vi "CSMOMgr-Create CSMO.vi"(7 "Allowed Messages(Empty for all)":string[](array[string]), 8 "error in (no error)":errorcluster, 10 "Name(\"\" to use uuid) in":string, 11 "CSMOMgr":T1) -> (0 "error out":errorcluster, 2 "CSMO":T2, 3 "CSMOMgr out":T1)   [LabVIEW 2020, in "Communicable State Machine.lvlib"]
uses:
  Communicable State Machine.lvlib
  Def-CSMOMgr.ctl
  _CSMObj.ctl
  Priority Queue.lvclass
  _CSM_MODE.ctl
  _CSMObj-Data.ctl
  _CSM Status Change Event Data.ctl
  _CSMObj-ModeData.ctl
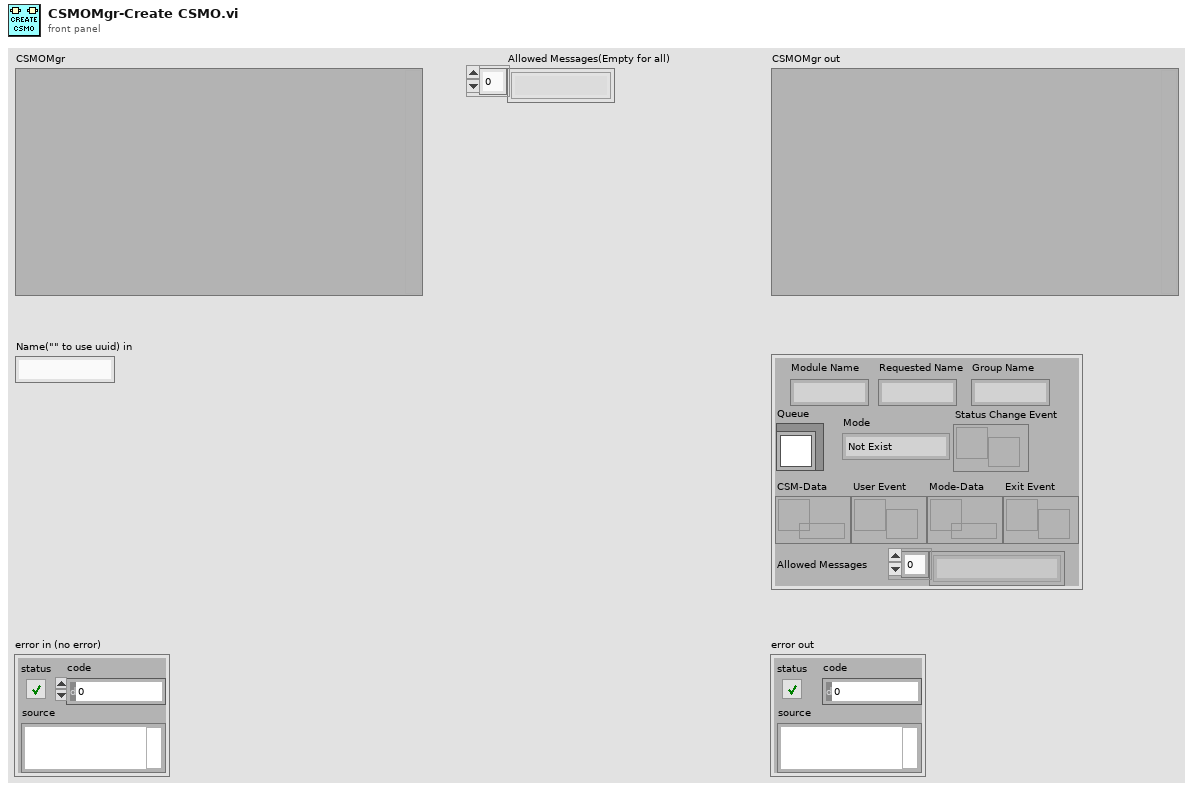
[diagram p1: front panel]
types:
  T1 = typedef "Communicable State Machine.lvlib/Def-CSMOMgr.ctl" = variant
  T2 = typedef "Communicable State Machine.lvlib/_CSMObj.ctl" = cluster{"Requested Name":string, "Module Name":string, "Mode":T3, "Queue":refnum<class "Priority Queue.lvclass">, "CSM-Data":refnum<data-value>, "User Event":refnum<user-event>, "Status Change Event":refnum<user-event>, "Allowed Messages":string[], "Mode-Data":refnum<data-value>, "Group Name":string, "Exit Event":refnum<user-event>}
  T3 = typedef "Communicable State Machine.lvlib/_CSM_MODE.ctl" = enum16{"Not Exist", "Stand Alone", "CSM", "Worker Agent", "Worker", "Chain", "Chain Node"}
  T4 = typedef "Communicable State Machine.lvlib/_CSM_NAME_REQUEST.ctl" = enum16{"Stand Alone CSM Request", "Normal CSM Request", "Agent Request", "Action Worker Request", "Chain Request", "Chain Node Request"}
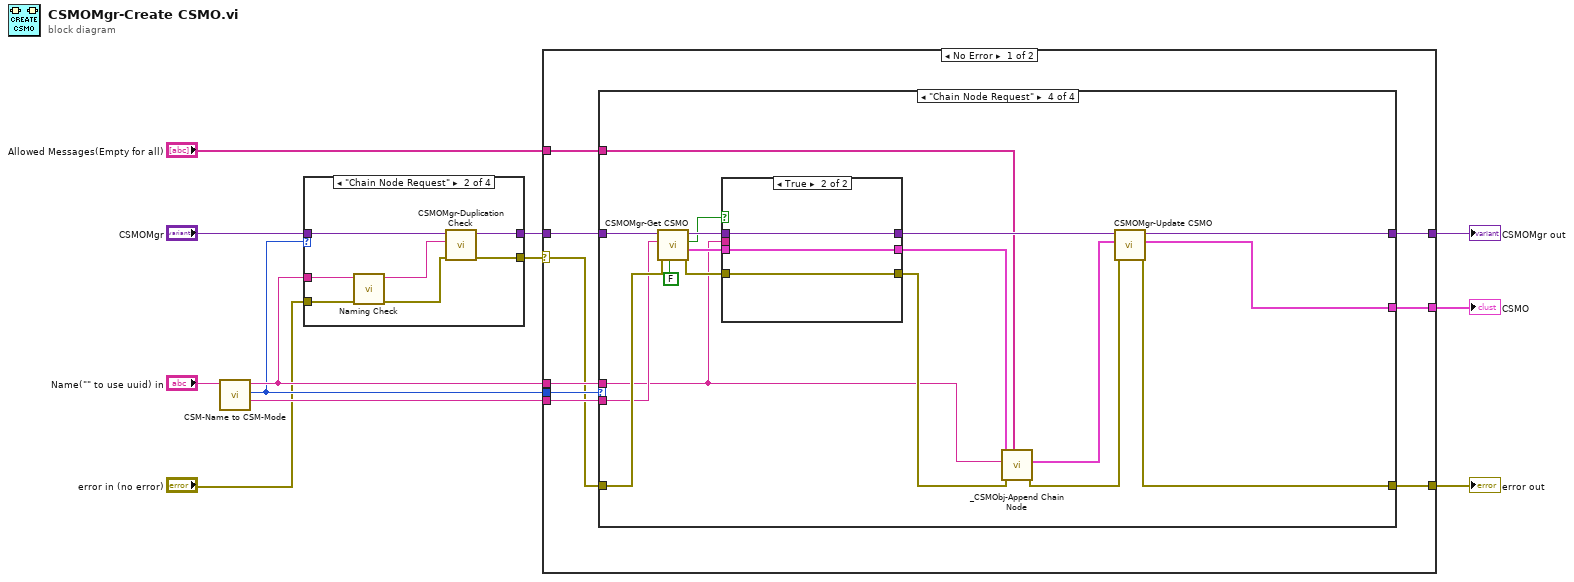
[diagram p0: block diagram]
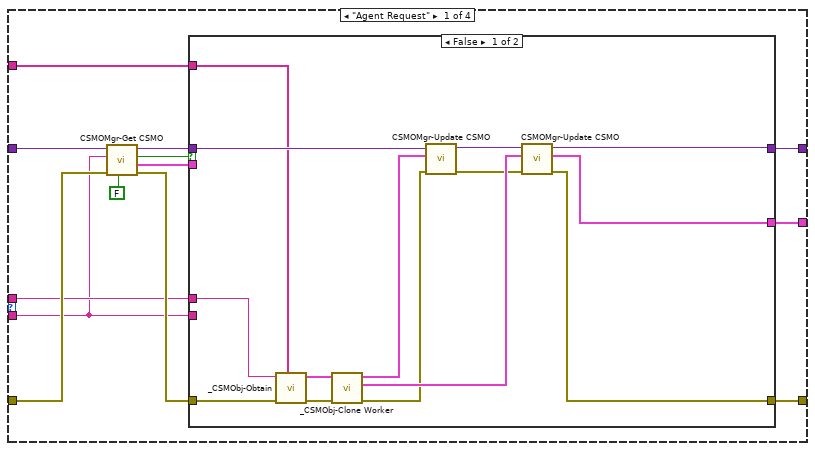
[diagram p2: hidden frame]
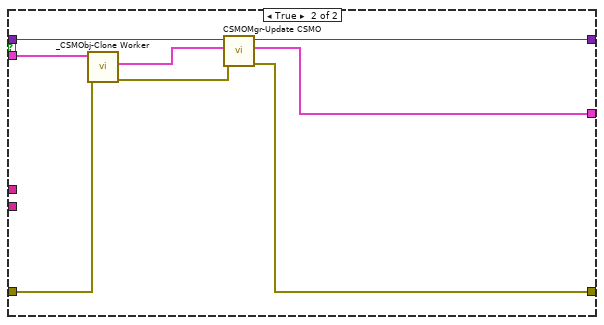
[diagram p3: hidden frame]
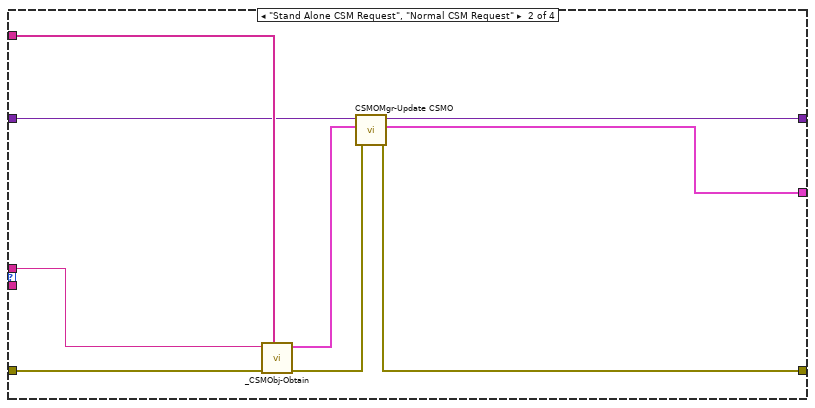
[diagram p4: hidden frame]
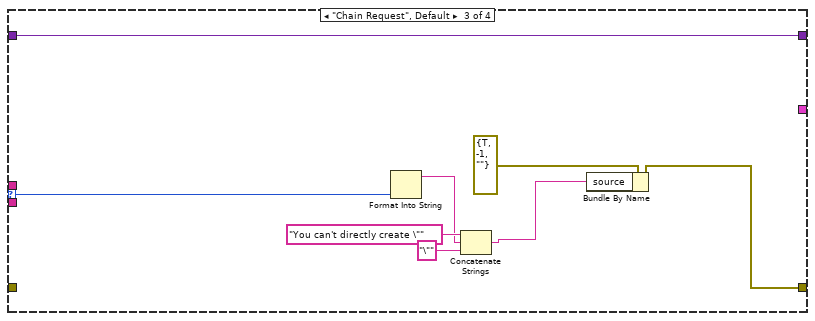
[diagram p5: hidden frame]
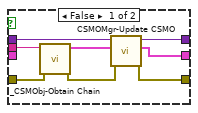
[diagram p6: hidden frame]
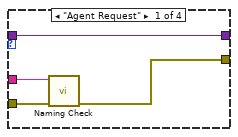
[diagram p8: hidden frame]
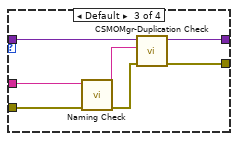
[diagram p9: hidden frame]
diagram:
  n1 = call "CSM-Name to CSM-Mode.vi"("String"="Name(\"\" to use uuid) in") -> ("ParentCSM Name"=w10:string, "CSM Mode"=w11:T4, "Requested Name"=w12:string)  [unwired: 8 in]
  n2 = case shown="\"Chain Node Request\"" w11 {
    tunnel: [w14 w20 w30 w32] -> w6
    tunnel: [w13 w18 w28 w31] -> w7
    tunnel: "CSMOMgr" -> [w14 w21 w26 w32]
    tunnel: "error in (no error)" -> [w15 w22 w25 w31]
    tunnel: w12 -> [w16 w23 w24 _]
    frame "Agent Request" {
      n3 = call "Naming Check.vi"("error in (no error)"=w15, "Name(\"\" to use uuid)"=w16) -> ("error out"=w13:errorcluster)  [unwired: 8 in, 1 out]
    }
    frame "Chain Node Request" {
      n4 = call "Naming Check.vi"("error in (no error)"=w22, "Name(\"\" to use uuid)"=w23) -> ("error out"=w17:errorcluster, "Name(dup)"=w19:string)  [unwired: 8 in]
      n5 = call "CSMOMgr-Duplication Check.vi"("Error in"=w17, "Queue Name"=w19, "CSMOMgr"=w21) -> ("Error out"=w18:errorcluster, "CSMOMgr out"=w20:T1)  [unwired: 7 in]
    }
    frame Default {
      n6 = call "Naming Check.vi"("error in (no error)"=w25, "Name(\"\" to use uuid)"=w24) -> ("error out"=w29:errorcluster, "Name(dup)"=w27:string)  [unwired: 8 in]
      n7 = call "CSMOMgr-Duplication Check.vi"("Error in"=w29, "Queue Name"=w27, "CSMOMgr"=w26) -> ("Error out"=w28:errorcluster, "CSMOMgr out"=w30:T1)  [unwired: 7 in]
    }
    frame "Stand Alone CSM Request" {
    }
  }
  n8 = case shown="No Error" w7 {
    selector: w7 -> [w38 w124]
    tunnel: w12 -> [w41 _]
    tunnel: w11 -> [w40 _]
    tunnel: w10 -> [w39 _]
    tunnel: w6 -> [w37 w123]
    tunnel: "Allowed Messages(Empty for all)" -> [w36 _]
    tunnel: [w35 w124] -> w3
    tunnel: [w34 w123] -> w2
    tunnel: [w33 _] -> w1
    frame No Error {
      n9 = case shown="\"Chain Node Request\"" w40 {
        selector: w40 -> [_ _ w89 _]
        tunnel: [w54 w85 w93 w101] -> w34
        tunnel: [w53 w84 w87 w97] -> w35
        tunnel: w36 -> [w52 w83 _ w96]
        tunnel: [w51 w78 _ w99] -> w33
        tunnel: w37 -> [w47 w82 w93 w110]
        tunnel: w38 -> [w46 w81 _ w109]
        tunnel: w41 -> [w43 w80 _ w94]
        tunnel: w39 -> [w42 _ _ w108]
        frame "Agent Request" {
          n10 = call "CSMOMgr-Get CSMO.vi"("GenError?(T)"=FALSE, "Error in"=w46, "Queue Name"=w42, "CSMOMgr"=w47) -> ("Error out"=w48:errorcluster, "values"=w49:T2, "found"=w45:bool, "CSMOMgr out"=w50:T1)  [unwired: 4 in]
          n11 = case shown="False" w45 {
            tunnel: [w56 w69] -> w51
            tunnel: w50 -> [w68 w73]
            tunnel: [w63 w72] -> w54
            tunnel: w49 -> [_ w76]
            tunnel: w48 -> [w67 w75]
            tunnel: [w57 w70] -> w53
            tunnel: w43 -> [w55 _]
            tunnel: w52 -> [w66 _]
            tunnel: w42 -> [_ _]
            frame False {
              n12 = call "_CSMObj-Obtain.vi"("Allowed Messages(Empty for all)"=w66, "Error in"=w67, "Requested Name"=w55) -> ("Error out"=w61:errorcluster, "CSMQ out"=w65:T2)  [unwired: 7 in]
              n13 = call "_CSMObj-Clone Worker.vi"("Error in"=w61, "CSMObj in"=w65) -> ("Error out"=w59:errorcluster, "output cluster"=w62:T2, "CSMObj out"=w60:T2)  [unwired: 7 in]
              n14 = call "CSMOMgr-Update CSMO.vi"("error in (no error)"=w59, "CSMO"=w60, "CSMOMgr in"=w68) -> ("error out"=w58:errorcluster, "CSMOMgr out"=w64:T1)  [unwired: 6 in, 1 out]
              n15 = call "CSMOMgr-Update CSMO.vi"("error in (no error)"=w58, "CSMO"=w62, "CSMOMgr in"=w64) -> ("error out"=w57:errorcluster, "CSMO(dup)"=w56:T2, "CSMOMgr out"=w63:T1)  [unwired: 6 in]
            }
            frame True {
              n16 = call "_CSMObj-Clone Worker.vi"("Error in"=w75, "CSMObj in"=w76) -> ("Error out"=w71:errorcluster, "output cluster"=w74:T2)  [unwired: 7 in, 1 out]
              n17 = call "CSMOMgr-Update CSMO.vi"("error in (no error)"=w71, "CSMO"=w74, "CSMOMgr in"=w73) -> ("error out"=w70:errorcluster, "CSMO(dup)"=w69:T2, "CSMOMgr out"=w72:T1)  [unwired: 6 in]
            }
          }
        }
        frame "Stand Alone CSM Request", "Normal CSM Request" {
          n18 = call "_CSMObj-Obtain.vi"("Allowed Messages(Empty for all)"=w83, "Error in"=w81, "Requested Name"=w80) -> ("Error out"=w79:errorcluster, "CSMQ out"=w77:T2)  [unwired: 7 in]
          n19 = call "CSMOMgr-Update CSMO.vi"("error in (no error)"=w79, "CSMO"=w77, "CSMOMgr in"=w82) -> ("error out"=w84:errorcluster, "CSMO(dup)"=w78:T2, "CSMOMgr out"=w85:T1)  [unwired: 6 in]
        }
        frame "Chain Request", Default {
          n20 = Format Into String(w89) -> (resulting string=w88:string)  [unwired: 3 in, 1 out]
          n21 = Concatenate Strings("You can't directly create \"" ("source"), w88, "\"" ("source")) -> (w86:string)
          n22 = Bundle By Name(cluster=errorcluster {"status"=TRUE, "code"=-1, "source"=""} ("error out"), "source"=w86) -> (w87:errorcluster)
        }
        frame "Chain Node Request" {
          n23 = call "CSMOMgr-Get CSMO.vi"("GenError?(T)"=FALSE, "Error in"=w109, "Queue Name"=w108, "CSMOMgr"=w110) -> ("Error out"=w107:errorcluster, "values"=w105:T2, "found"=w104:bool, "CSMOMgr out"=w106:T1)  [unwired: 4 in]
          n24 = case shown="True" w104 {
            tunnel: w94 -> [w119 _]
            tunnel: w107 -> [w118 w121]
            tunnel: [w117 w121] -> w95
            tunnel: w106 -> [w116 w120]
            tunnel: w105 -> [_ w122]
            tunnel: [w113 w122] -> w103
            tunnel: [w112 w120] -> w102
            frame False {
              n25 = call "_CSMObj-Obtain Chain.vi"("Error in"=w118, "Requested Name"=w119) -> ("Error out"=w115:errorcluster, "CSMQ out"=w114:T2)  [unwired: 8 in]
              n26 = call "CSMOMgr-Update CSMO.vi"("error in (no error)"=w115, "CSMO"=w114, "CSMOMgr in"=w116) -> ("error out"=w117:errorcluster, "CSMO(dup)"=w113:T2, "CSMOMgr out"=w112:T1)  [unwired: 6 in]
            }
            frame True {
            }
          }
          n27 = call "_CSMObj-Append Chain Node.vi"("Allowed Messages(Empty for all)"=w96, "Error in"=w95, "Requested Name"=w94, "CSMObj in"=w103) -> ("Error out"=w98:errorcluster, "output cluster (dup)"=w100:T2)  [unwired: 5 in, 1 out]
          n28 = call "CSMOMgr-Update CSMO.vi"("error in (no error)"=w98, "CSMO"=w100, "CSMOMgr in"=w102) -> ("error out"=w97:errorcluster, "CSMO(dup)"=w99:T2, "CSMOMgr out"=w101:T1)  [unwired: 6 in]
        }
      }
    }
    frame Error {
    }
  }
  "CSMO" <- w1
  "error out" <- w3
  "CSMOMgr out" <- w2
